vi "set_General_p.vi"(0 "MoAgSy_Host":refnum<class "MoAgSy_Host.lvclass">, 2 "General":T1, 5 "error in (no error)":errorcluster) -> (14 "dup MoAgSy_Host":refnum<class "MoAgSy_Host.lvclass">, 19 "error out":errorcluster)   [LabVIEW 2009, in "MoAgSy.lvlib" / "MoAgSy_Host.lvclass"]
doc: "<B>protected</B> VI sets general settings of mobile agent host class.\nIs called by public set general settings VI and during host creation process\n\nF.Berck@gsi.de\nGSI Darmstadt 2009"
uses:
  MoAgSy_Host.lvclass
  MoAgSy_Host.lvclass/MoAgSy_Host.ctl
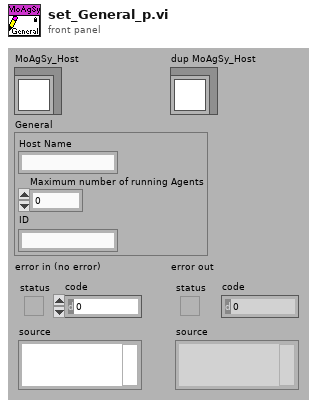
[diagram p1: front panel]
types:
  T1 = cluster{"Host Name":string, "Maximum number of running Agents":i16, "ID":string}
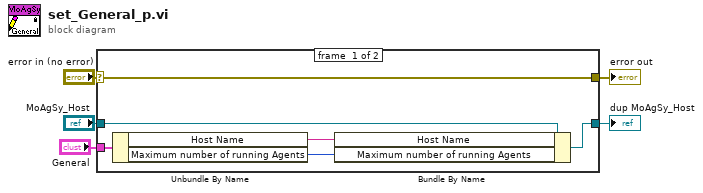
[diagram p0: block diagram]
diagram:
  n1 = case shown="No Error" "error in (no error)" {
    selector: "error in (no error)" -> [w11 w12]
    tunnel: [w11 w12] -> w4
    tunnel: [w9 w13] -> w2
    tunnel: "MoAgSy_Host" -> [w10 w13]
    tunnel: "General" -> [w8 _]
    frame #0 {
      n2 = Unbundle By Name(w8) -> ("Host Name"=w6:string, "Maximum number of running Agents"=w7:i16)
      n3 = Bundle By Name(cluster=w10, "Host Name"=w6, "Maximum number of running Agents"=w7) -> (w9:refnum<class "MoAgSy_Host.lvclass">)
    }
    frame #1 {
    }
  }
  "error out" <- w4
  "dup MoAgSy_Host" <- w2
